vi "isCached.vi"(8 "error in (no error)":errorcluster, 10 "Topic":string, 11 "TopicFilter in":refnum<class "TopicFilter.lvclass">) -> (0 "error out":errorcluster, 1 "found?":bool, 2 "Topic dup":string, 3 "TopicFilter out":refnum<class "TopicFilter.lvclass">)   [LabVIEW 2013, in "MQTT Base.lvlib" / "TopicFilter.lvclass"]
uses:
  TopicFilter.lvclass
  TopicFilter.lvclass/TopicFilter.ctl
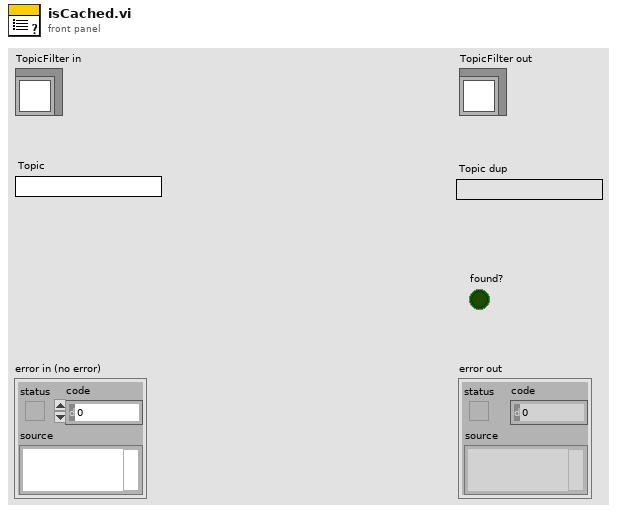
[diagram p1: front panel]
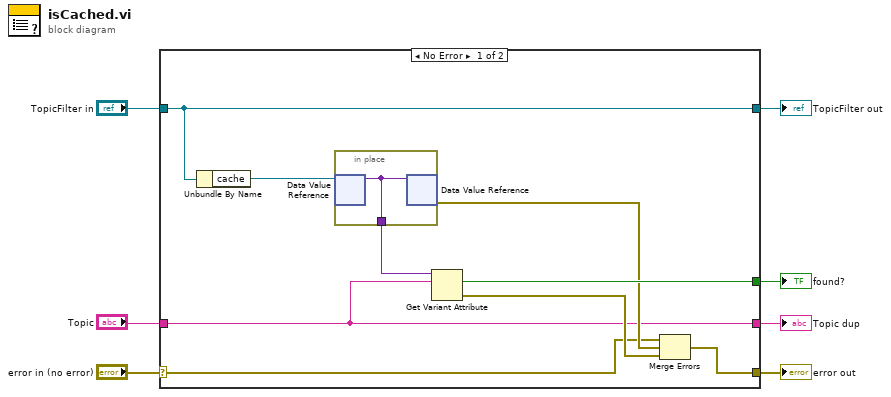
[diagram p0: block diagram]
diagram:
  n1 = case shown="No Error" "error in (no error)" {
    selector: "error in (no error)" -> [w10 w20]
    tunnel: [w9 w20] -> w6
    tunnel: [w13 w19] -> w4
    tunnel: "TopicFilter in" -> [w13 w19]
    tunnel: "Topic" -> [w8 w18]
    tunnel: [w15 _] -> w2
    tunnel: [w8 w18] -> w1
    frame No Error {
      n2 = Unbundle By Name(w13) -> ("cache"=w12:refnum<data-value>)
      n3 = in-place {
        in-place-border: [w17] -> w16
        n4 = in-place-dvr #1(w12) -> (w17:variant)  [unwired: 1 out]
        n5 = in-place-dvr #1(w17) -> (w14:errorcluster)  [unwired: 1 out]
      }
      n6 = Get Variant Attribute(Variant=w16, name=w8) -> (found=w15:bool, error out=w11:errorcluster)  [unwired: 2 in, 2 out]
      n7 = Merge Errors(w10, w14, w11) -> (w9:errorcluster)
    }
    frame Error {
    }
  }
  "error out" <- w6
  "TopicFilter out" <- w4
  "found?" <- w2
  "Topic dup" <- w1
